vi "PresetWrist.vi"(11 "Cluster":T1={"Drive Forward Input "=0.0, "Drive Twist Input"=0.0, "Drive Output"=0.0, "Drivetwist Output"=0.0, "Left Joystick Buttons"=[], "Left Joystick Axis"=[], "Right Joystick Axis"=[-0.007874015748031496, 0.0, -0.10236220472440945, -0.6771653543307087], "Right Joystick Button"=[FALSE, FALSE, FALSE, FALSE, FALSE, FALSE, FALSE, FALSE, FALSE, FALSE, FALSE, FALSE], "Arm Encoder"=0.0, "Left Drive Encoder"=5282.0, "Right Drive Encoder"=5266.0, "Gyro Angle "=0.0, "Arm Joystick Output  "=0.0, "Line Follower L, C, R "=[TRUE, TRUE, TRUE], "Line follow?"=FALSE, " Climb Solenoid"=FALSE, "Wrist Encoder Count"=0.0, "Wrist Joystick Output"=0.0, "Ball Encoder Count"=0.0, "Ball Output"=0.0, "Climb Encoder"=0.0, "Climb Motor Output"=0.0, " Hatch Solenoid"=FALSE, "Arm Setpoint "=4.0, "Wrist Setpoint "=0.0, "Arm Joystick Enabled?"=FALSE, "Wrist Joystick Enabled"=FALSE, "Vision String"="", "Left Joystick POVs"=[]}) -> (3 "Numeric":dbl=6.0 format="%#_13g")   [LabVIEW 2018]
uses:
  TypeDefs/Teleop Data Cluster.ctl
  TypeDefs/Joystick Buttons.ctl
panel:
  in  "Lookup Table 2":dbl[](array[numeric])=[0.0, 1.0, 2.0, 0.0, 0.0, 1.0]
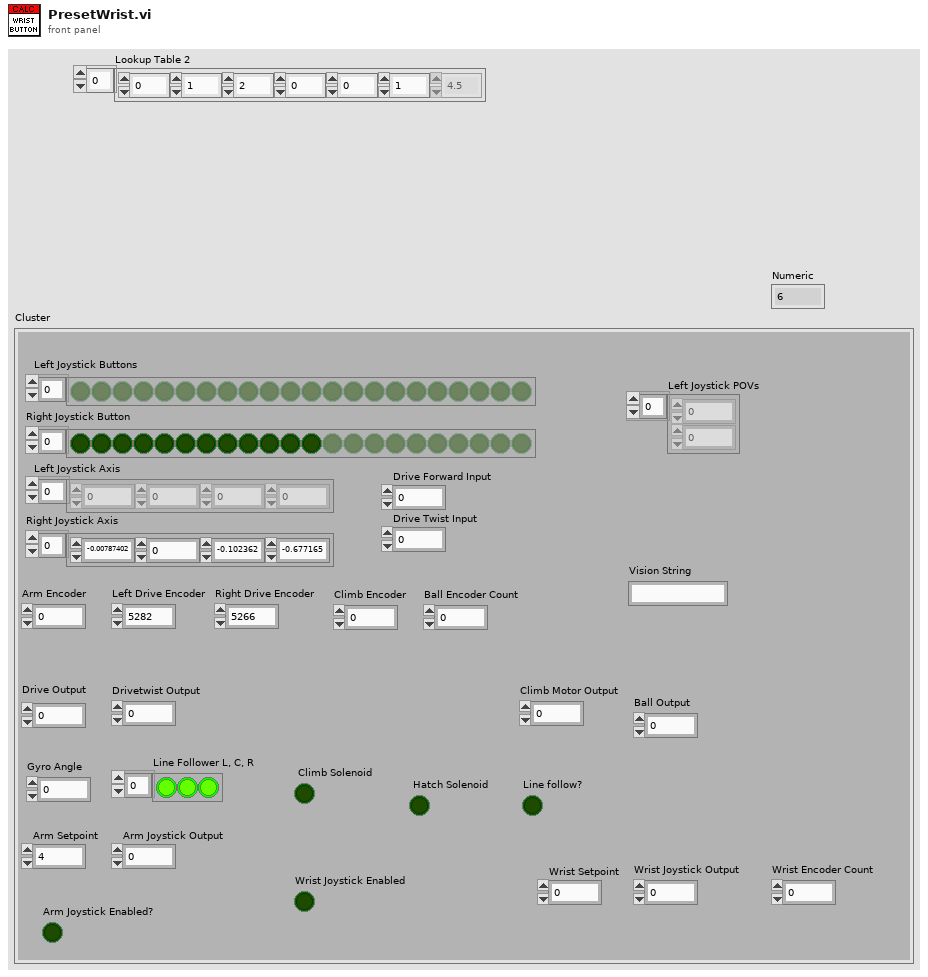
[diagram p1: front panel]
types:
  T1 = typedef "Teleop Data Cluster.ctl" = cluster{"Drive Forward Input ":dbl, "Drive Twist Input":dbl, "Drive Output":dbl, "Drivetwist Output":dbl, "Left Joystick Buttons":bool[], "Left Joystick Axis":dbl[], "Right Joystick Axis":dbl[], "Right Joystick Button":bool[], "Arm Encoder":dbl, "Left Drive Encoder":dbl, "Right Drive Encoder":dbl, "Gyro Angle ":dbl, "Arm Joystick Output  ":dbl, "Line Follower L, C, R ":bool[], "Line follow?":bool, " Climb Solenoid":bool, "Wrist Encoder Count":dbl, "Wrist Joystick Output":dbl, "Ball Encoder Count":dbl, "Ball Output":dbl, "Climb Encoder":dbl, "Climb Motor Output":dbl, " Hatch Solenoid":bool, "Arm Setpoint ":dbl, "Wrist Setpoint ":dbl, "Arm Joystick Enabled?":bool, "Wrist Joystick Enabled":bool, "Vision String":string, "Left Joystick POVs":i16[]}
  T2 = typedef "Joystick Buttons.ctl" = enum16{"Trigger", "Thumb", "Top 3", "Top 4", "Top 5", "Top 6", "Bottom 7", "Bottom 8", "Bottom 9", "Bottom 10", "Bottom 11", "Bottom 12"}
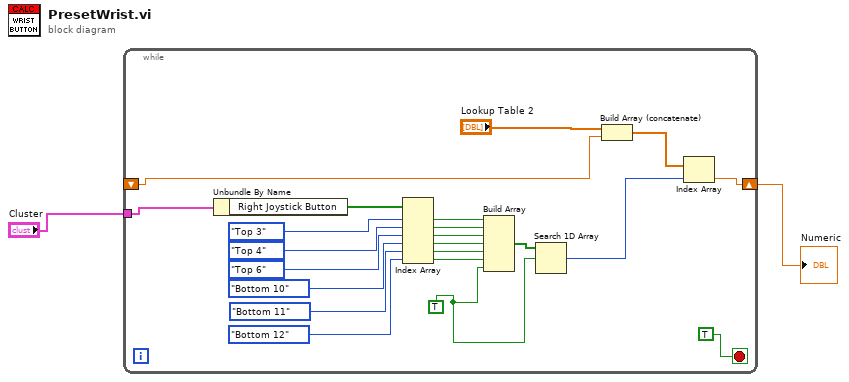
[diagram p0: block diagram]
diagram:
  n1 = while {
    shift-right: [w5] -> w2
    shift-left: _ -> [w6]
    tunnel: "Cluster" -> [w7]
    stop <- TRUE stop-if-true
    w4 = TRUE ("element")
    n2 = Unbundle By Name(w7) -> ("Right Joystick Button"=w24:bool[])
    n3 = Index Array(array=w24, index #1=Joystick_Buttons."Top 3" ("Enum"), index #2=Joystick_Buttons."Top 4" ("Enum"), index #3=Joystick_Buttons."Top 6" ("Enum"), index #4=Joystick_Buttons."Bottom 10" ("Enum"), index #5=Joystick_Buttons."Bottom 11" ("Enum"), index #6=Joystick_Buttons."Bottom 12" ("Enum")) -> (element #1=w19:bool, element #2=w18:bool, element #3=w17:bool, element #4=w16:bool, element #5=w9:bool, element #6=w8:bool)
    n4 = Build Array(w19, w18, w17, w16, w9, w8, w4) -> (w15:bool[])
    n5 = Search 1D Array(1D array=w15, element=w4) -> (index of element=w14:i32)  [unwired: 1 in]
    n6 = Build Array (concatenate)("Lookup Table 2", w6) -> (w12:dbl[])
    n7 = Index Array(array=w12, index=w14) -> (element=w5:dbl)
  }
  "Numeric" <- w2
